vi "PhotonPipelineResult_GetMetadata.vi"(11 "PhotonPipelineResult":T2={"Targets"=[], "PhotonMultiTargetPNPResult"={"PhotonPNPResult"={"IsPresent"=FALSE, "bestReprojErr"=0.0, "altReprojErr"=0.0, "ambiguity"=0.0, "Best"={"TRANSLATION3D"={"X"=0.0, "Y"=0.0, "Z"=0.0}, "ROTATION3D"={"Q_quaternion"={"R"=1.0, "V"=[0.0, 0.0, 0.0]}}, "XF"=FALSE}, "Alt"={"TRANSLATION3D"={"X"=0.0, "Y"=0.0, "Z"=0.0}, "ROTATION3D"={"Q_quaternion"={"R"=1.0, "V"=[0.0, 0.0, 0.0]}}, "XF"=FALSE}}, "FiducialIDsUsed"=[]}, "PhotonPipelineMetadata"={"CaptureTimestampMicros"=0, "PublishTimestampMicros"=0, "SequenceID"=0, "TimeSinceLastPong"=0}} {"PhotonMultiTargetPNPResult"."PhotonPNPResult"."Alt"."TRANSLATION3D"."Z" format="%14.3f"; "PhotonMultiTargetPNPResult"."PhotonPNPResult"."Alt"."TRANSLATION3D"."Y" format="%14.3f"; "PhotonMultiTargetPNPResult"."PhotonPNPResult"."Alt"."TRANSLATION3D"."X" format="%14.3f"; "PhotonMultiTargetPNPResult"."PhotonPNPResult"."Best"."TRANSLATION3D"."Z" format="%14.3f"; "PhotonMultiTargetPNPResult"."PhotonPNPResult"."Best"."TRANSLATION3D"."Y" format="%14.3f"; "PhotonMultiTargetPNPResult"."PhotonPNPResult"."Best"."TRANSLATION3D"."X" format="%14.3f"; "Targets"."AltCameraToTarget"."TRANSLATION3D"."Z" format="%14.3f"; "Targets"."AltCameraToTarget"."TRANSLATION3D"."Y" format="%14.3f"; "Targets"."AltCameraToTarget"."TRANSLATION3D"."X" format="%14.3f"; "Targets"."BestCameraToTarget"."TRANSLATION3D"."Z" format="%14.3f"; "Targets"."BestCameraToTarget"."TRANSLATION3D"."Y" format="%14.3f"; "Targets"."BestCameraToTarget"."TRANSLATION3D"."X" format="%14.3f"}) -> (3 "PipelineMetadata":T1)   [LabVIEW 2019, in "PhotonVisionLib.lvlib"]
doc: "Returns the metadata in this pipeline result. \nInputs:\n - PipelineResult -- Parsed PipelineResult cluster.\n\nOutputs:\n - Metadata -- Metadata cluster."
uses:
  TypeDef/PhotonPipelineResultType.ctl
  TypeDef/PhotonTrackedTargetType.ctl
  TypeDef/TargetCornerType.ctl
  <vilib>/Rock Robotics/WPI/ThirdParty/JAS_Junk/TrajLib/TypeDef/TRANSFORM3D.ctl
  <vilib>/Rock Robotics/WPI/ThirdParty/JAS_Junk/TrajLib/TypeDef/TRANSLATION3D.ctl
  <vilib>/Rock Robotics/WPI/ThirdParty/JAS_Junk/TrajLib/TypeDef/ROTATION3D.ctl
  <vilib>/Rock Robotics/WPI/ThirdParty/JAS_Junk/TrajLib/TypeDef/QUATERNION.ctl
  TypeDef/PhotonMultiTargetPNPResultType.ctl
  TypeDef/PhotonPNPResultType.ctl
  TypeDef/PhotonPipelineMetadataType.ctl
  PhotonVisionLib.lvlib
  <vilib>/Rock Robotics/WPI/ThirdParty/JAS_Junk/TrajLib/Trajectory_Library.lvlib
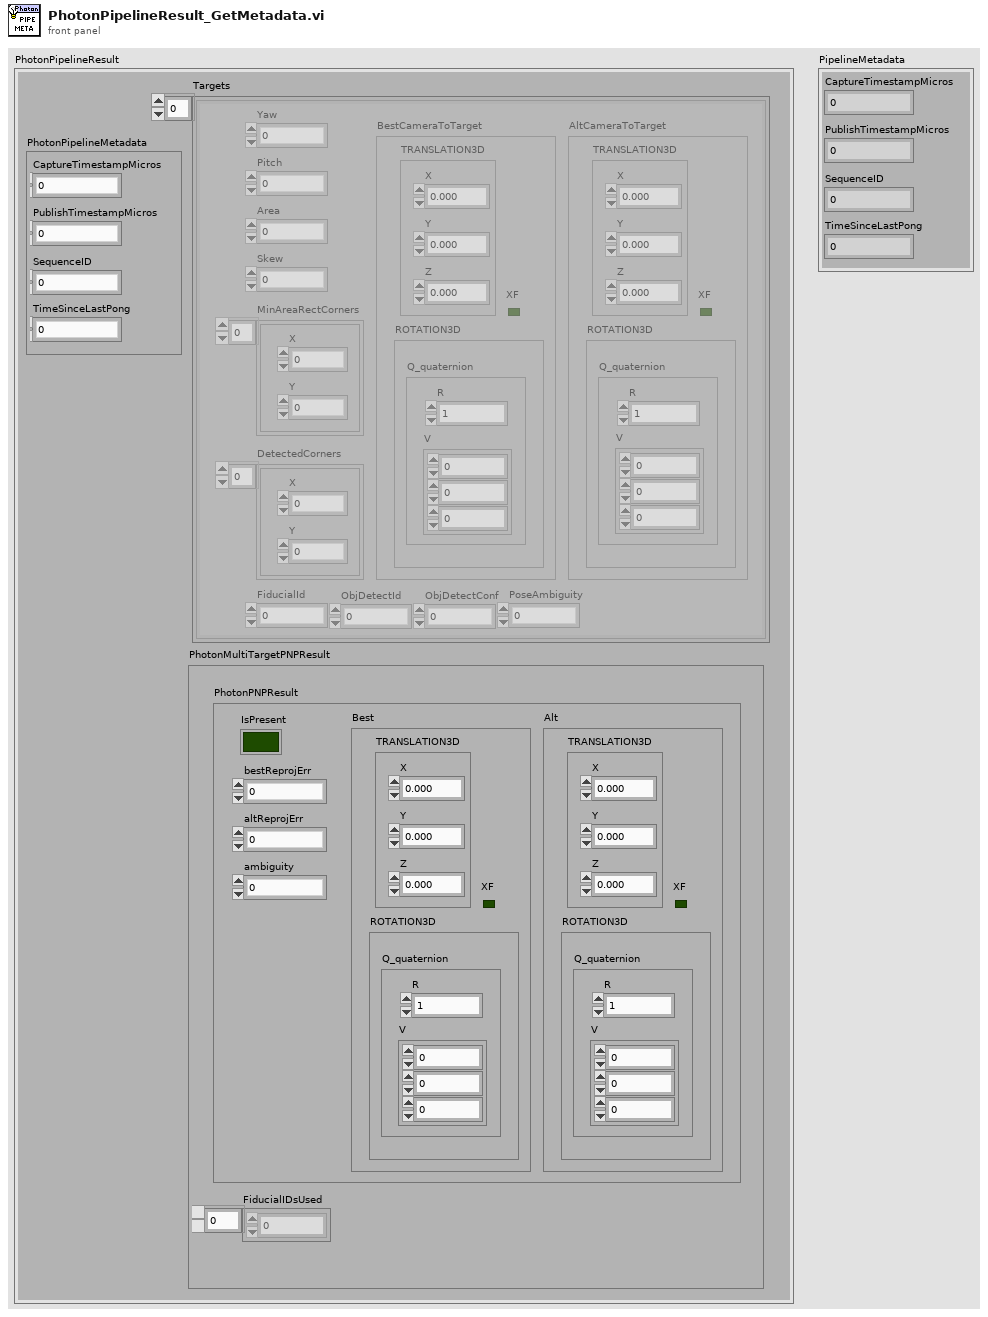
[diagram p1: front panel]
types:
  T1 = typedef "PhotonVisionLib.lvlib/PhotonPipelineMetadataType.ctl" = cluster{"CaptureTimestampMicros":i64, "PublishTimestampMicros":i64, "SequenceID":i64, "TimeSinceLastPong":i64}
  T2 = typedef "PhotonVisionLib.lvlib/PhotonPipelineResultType.ctl" = cluster{"Targets":T3[], "PhotonMultiTargetPNPResult":T9, "PhotonPipelineMetadata":T1}
  T3 = typedef "PhotonVisionLib.lvlib/PhotonTrackedTargetType.ctl" = cluster{"Yaw":dbl, "Pitch":dbl, "Area":dbl, "Skew":dbl, "MinAreaRectCorners":T4[], "BestCameraToTarget":T5, "FiducialId":i32, "AltCameraToTarget":T5, "PoseAmbiguity":dbl, "DetectedCorners":T4[], "ObjDetectId":i32, "ObjDetectConf":sgl}
  T4 = typedef "PhotonVisionLib.lvlib/TargetCornerType.ctl" = cluster{"X":dbl, "Y":dbl}
  T5 = typedef "Trajectory_Library.lvlib/TRANSFORM3D.ctl" = cluster{"TRANSLATION3D":T6, "ROTATION3D":T7, "XF":bool}
  T6 = typedef "Trajectory_Library.lvlib/TRANSLATION3D.ctl" = cluster{"X":dbl, "Y":dbl, "Z":dbl}
  T7 = typedef "Trajectory_Library.lvlib/ROTATION3D.ctl" = cluster{"Q_quaternion":T8}
  T8 = typedef "Trajectory_Library.lvlib/QUATERNION.ctl" = cluster{"R":dbl, "V":dbl[]}
  T9 = typedef "PhotonVisionLib.lvlib/PhotonMultiTargetPNPResultType.ctl" = cluster{"PhotonPNPResult":T10, "FiducialIDsUsed":i16[]}
  T10 = typedef "PhotonVisionLib.lvlib/PhotonPNPResultType.ctl" = cluster{"IsPresent":bool, "bestReprojErr":dbl, "altReprojErr":dbl, "ambiguity":dbl, "Best":T5, "Alt":T5}
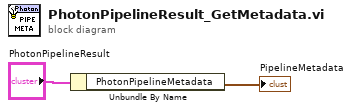
[diagram p0: block diagram]
diagram:
  n1 = Unbundle By Name("PhotonPipelineResult") -> ("PhotonPipelineMetadata"=→"PipelineMetadata":T1)
